vi "ClearBuffer.vi"(8 "error in (no error)":errorcluster caption="错误输入（无错误）", 9 "CANInd":u32, 10 "DeciceInd":u32, 11 "DeviceType":u32) -> (0 "error out":errorcluster caption="错误输出", 3 "Valid":bool)   [LabVIEW 2011]
uses:
  data/ControlCAN.dll
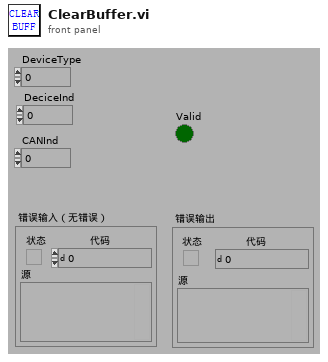
[diagram p1: front panel]
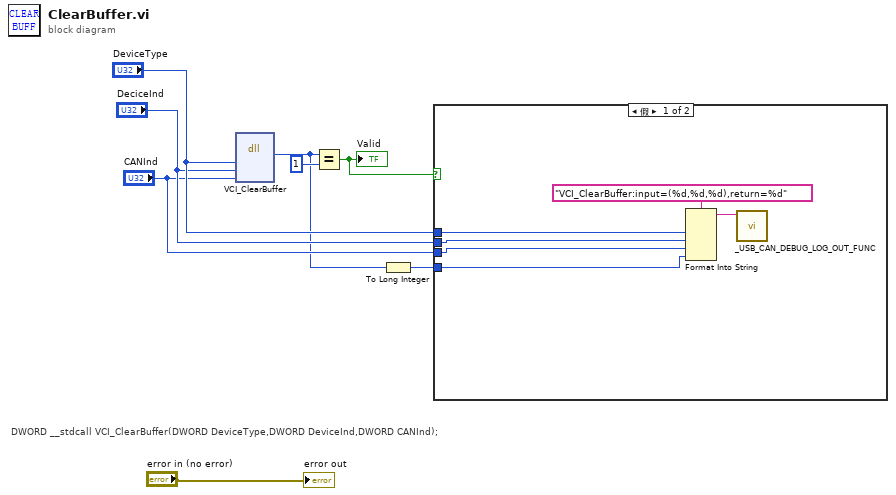
[diagram p0: block diagram]
diagram:
  # "DWORD __stdcall VCI_ClearBuffer(DWORD DeviceType,DWORD DeviceInd,DWORD CANInd);"
  n1 = dll-call lib="PTH1Mabs ZHost_E工作TnewcodeUSB CAN Tool1.97dataControlCAN.dll" fn="VCI_ClearBuffer"("DeviceType"="DeviceType", "DeciceInd"="DeciceInd", "CANInd"="CANInd") -> ("返回类型"=w2:u32)  [unwired: 6 in, 2 out]
  n2 = Equal?(x=w2, y=u32 1) -> (x = y?=w6:bool)
  "Valid" <- w6
  n3 = To Long Integer(number=w2) -> (32bit integer=w1:i32)
  n4 = case shown="假" w6 {
    tunnel: "DeviceType" -> [w12 _]
    tunnel: "DeciceInd" -> [w11 _]
    tunnel: "CANInd" -> [w10 _]
    tunnel: w1 -> [w9 _]
    frame False {
      n5 = Format Into String(format string="VCI_ClearBuffer:input=(%d,%d,%d),return=%d", w12, w11, w10, w9) -> (resulting string=w13:string)  [unwired: 2 in, 1 out]
      n6 = call "_USB_CAN_DEBUG_LOG_OUT_FUNC.vi"("Info"=w13) -> ()  [unwired: 11 in]
    }
    frame True {
    }
  }
  "error out" <- "error in (no error)"
